vi "Return To Null ClockWise.vi"(8 "错误输入（无错误）":errorcluster, 11 "VISA资源名称":refnum<visa-resource-name>) -> (0 "错误输出（无错误）":errorcluster caption="错误输入（无错误）", 3 "VISA资源名称":refnum<visa-resource-name>)   [LabVIEW 2015]
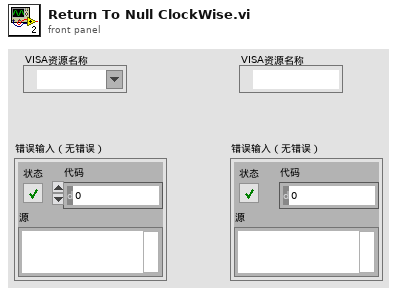
[diagram p1: front panel]
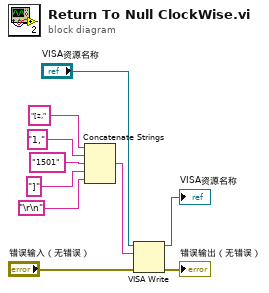
[diagram p0: block diagram]
diagram:
  n1 = Concatenate Strings("[z," ("字符串"), "1," ("字符串"), "1501" ("字符串"), "]" ("字符串"), "\r\n") -> (w4:string)
  n2 = VISA Write(VISA resource name="VISA资源名称", write buffer=w4, error in (no error)="错误输入（无错误）") -> (VISA resource name out=→"VISA资源名称":refnum<visa-resource-name>, error out=→"错误输出（无错误）":errorcluster)  [unwired: 1 out]
